vi "AlignTunnelsToControls.vi"(8 "Error In":errorcluster, 10 "New case structure ref":refnum<vi>, 11 "VI ref in":refnum<vi>) -> (0 "Error Out":errorcluster)   [LabVIEW 2017, in "ErrorStructureDrawer.lvlib"]
doc: "Aligns each tunnel on the new case structure to the control/indicator that it is wired to.\n\nNote that the case selector is not aligned by this VI."
uses:
  ErrorStructureDrawer.lvlib
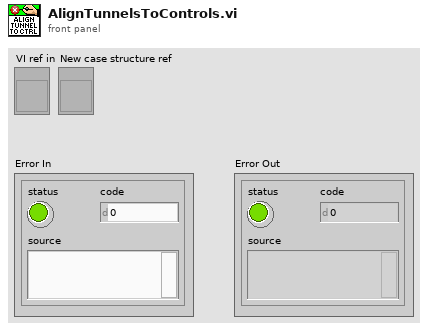
[diagram p1: front panel]
types:
  T1 = enum32{"LooseEnd", "Endpoint", "Bend", "Junction"}
  T2 = typedef "ErrorStructureDrawer.lvlib/ControlConstants.ctl" = cluster{"Half-height of terminal":i32}
  T3 = typedef "ErrorStructureDrawer.lvlib/CaseStructureConstants.ctl" = cluster{"Border thickness":u32, "Case-menu height":u32, "Half height/width of a tunnel":i32}
  T4 = cluster{"Position":cluster{"h":i16, "v":i16}, "Flags":i32, "Type":enum32{"LooseEnd", "Endpoint", "Bend", "Junction"}, "Up Joint Index":i16, "Down Joint Index":i16, "Left Joint Index":i16, "Right Joint Index":i16}[]
  T5 = cluster{"Position":cluster{"h":i16, "v":i16}, "Flags":i32, "Type":enum32{"LooseEnd", "Endpoint", "Bend", "Junction"}, "Up Joint Index":i16, "Down Joint Index":i16, "Left Joint Index":i16, "Right Joint Index":i16}
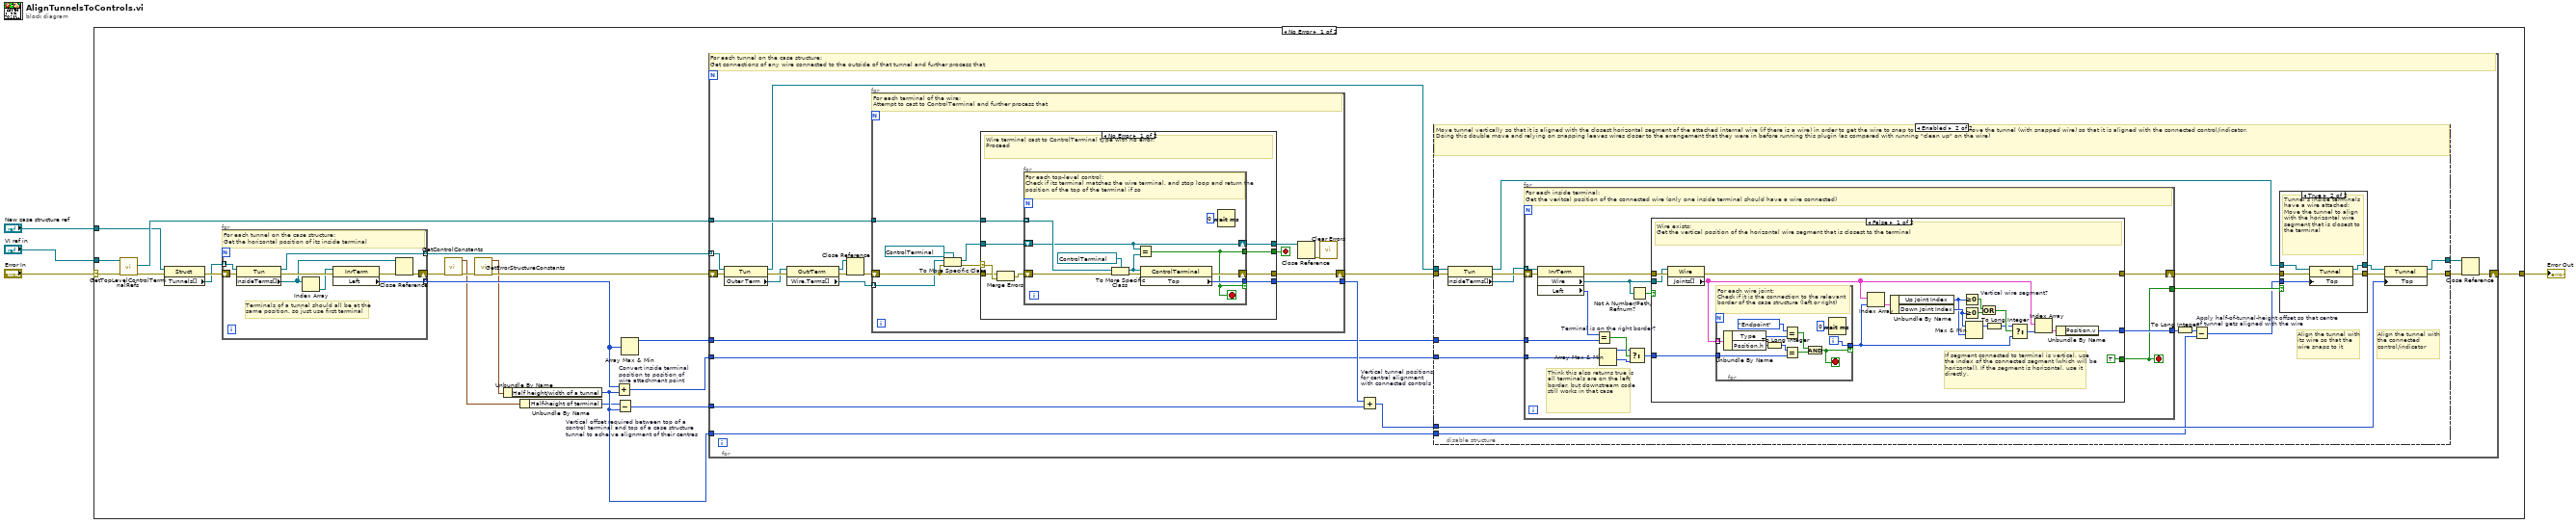
[diagram p0: block diagram]
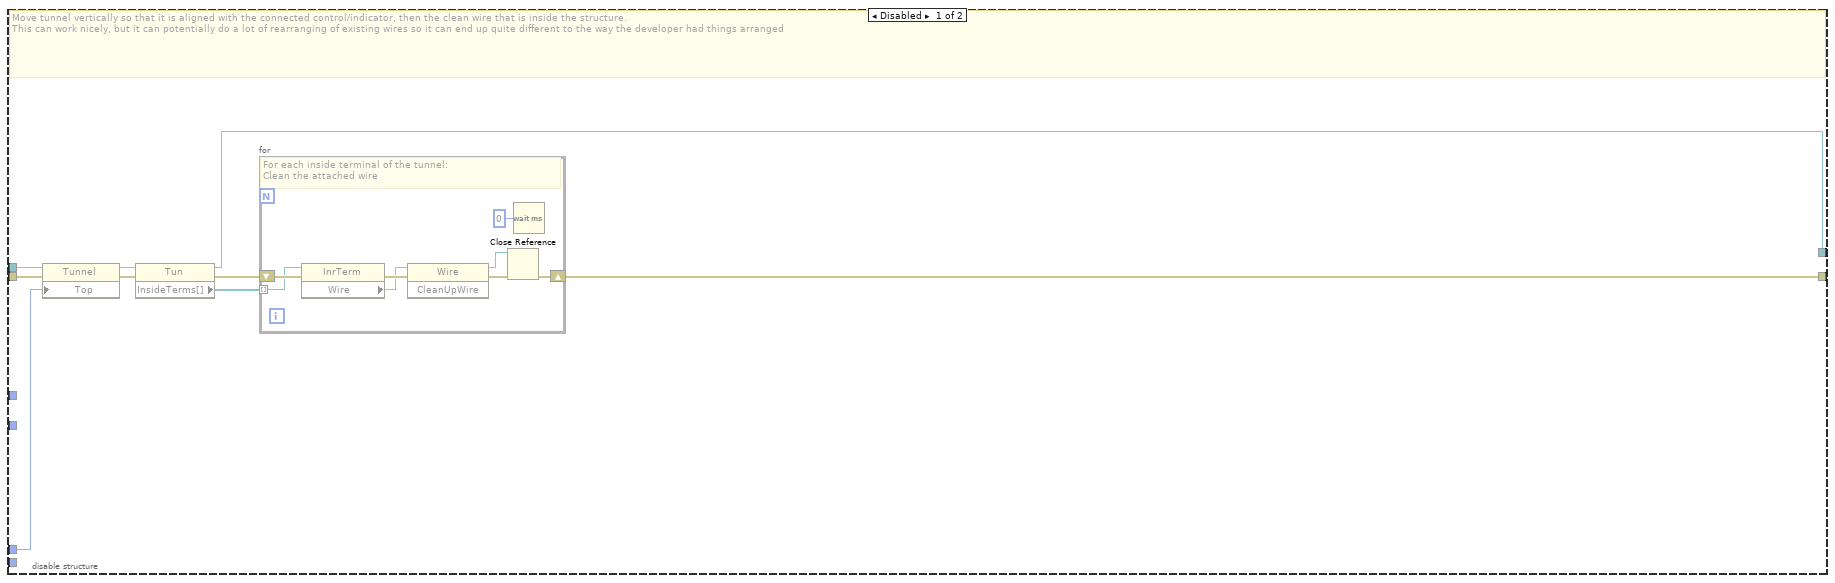
[diagram p2: hidden frame]
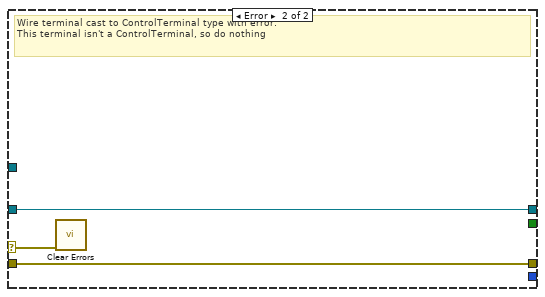
[diagram p5: hidden frame]
diagram:
  n1 = case shown="No Error" "Error In" {
    selector: "Error In" -> [w11 w174]
    tunnel: "VI ref in" -> [w20 _]
    tunnel: "New case structure ref" -> [w19 _]
    tunnel: [w10 w174] -> w1
    frame No Error {
      n2 = call "GetTopLevelControlTerminalRefs.vi"("error in (no error)"=w11, "VI ref in"=w20) -> ("error out"=w18:errorcluster, "Control terminals on top-level"=w21:refnum<vi>[])  [unwired: 7 in, 1 out]
      n3 = property class="Struct"(reference=w19, error in=w18) -> (error out=w22:errorcluster, "Tunnels[]"=w15:refnum<vi>[])  [unwired: 1 out]
      n4 = for {
        tunnel: w15 -> [w172] mode=indexing
        tunnel: [w170] -> w16 mode=indexing
        tunnel: [w169] -> w14 mode=indexing
        shift-right: [w165] -> w5
        shift-left: w22 -> [w168]
        # "Terminals of a tunnel should all be at the same position, so just use first terminal"
        # "For each tunnel on the case structure:\nGet the horizontal position of its inside terminal"
        n5 = property class="Tun"(reference=w172, error in=w168) -> (reference out=w169:refnum<vi>, error out=w173:errorcluster, "InsideTerms[]"=w167:refnum<vi>[])
        n6 = Index Array(array=w167) -> (element=w171:refnum<vi>)  [unwired: 1 in]
        n7 = property class="InrTerm"(reference=w171, error in=w173) -> (error out=w166:errorcluster, "Left"=w170:i32)  [unwired: 1 out]
        n8 = Close Reference(reference=w167, error in (no error)=w166) -> (error out=w165:errorcluster)
      }
      n9 = call "GetControlConstants.vi"("error in (no error)"=w5) -> ("error out"=w24:errorcluster, "Control constants"=w7:T2)  [unwired: 9 in]
      n10 = call "GetErrorStructureConstants.vi"("error in (no error)"=w24) -> ("error out"=w23:errorcluster, "Case structure constants"=w9:T3)  [unwired: 9 in]
      n11 = Unbundle By Name(w9) -> ("Half height/width of a tunnel"=w8:i32)
      n12 = Unbundle By Name(w7) -> ("Half-height of terminal"=w6:i32)
      n13 = Add "Convert inside terminal position to position of wire attachment point"(x=w16, y=w8) -> (x+y=w12:i32[])
      n14 = Subtract "Vertical offset required between top of a control terminal and top of a case structure tunnel to acheive alignment of their centres"(x=w6, y=w8) -> (x-y=w17:i32)
      n15 = Array Max & Min(array=w16) -> (max value=w13:i32)  [unwired: 3 out]
      n16 = for {
        tunnel: w14 -> [w43] mode=indexing
        tunnel: w21 -> [w42]
        shift-right: [w28] -> w10
        shift-left: w23 -> [w39]
        tunnel: w17 -> [w34]
        tunnel: w8 -> [w30]
        tunnel: w13 -> [w26]
        tunnel: w12 -> [w25]
        # "For each tunnel on the case structure:\nGet connections of any wire connected to the outside of that tunnel and further process that"
        n17 = property class="Tun"(reference=w43, error in=w39) -> (reference out=w31:refnum<vi>, error out=w44:errorcluster, "Outer Term"=w41:refnum<vi>)
        n18 = property class="OutrTerm"(reference=w41, error in=w44) -> (reference out=w37:refnum<vi>, error out=w38:errorcluster, "Wire.Terms[]"=w40:refnum<vi>[])
        n19 = Close Reference(reference=w37, error in (no error)=w38) -> (error out=w36:errorcluster)
        n20 = for {
          tunnel: w40 -> [w141] mode=indexing
          tunnel: w42 -> [w140]
          tunnel: [w139] -> w35
          shift-right: [w133] -> w32
          shift-left: w36 -> [w142]
          stop <- w138 stop-if-true
          # "For each terminal of the wire:\nAttempt to cast to ControlTerminal and further process that"
          n21 = To More Specific Class(target class=refnum<vi> refnum ("New case structure ref"), reference=w141, error in=w142) -> (specific class reference=w137:refnum<vi>, error out=w135:errorcluster)
          n22 = case shown="No Error" w135 {
            selector: w135 -> [w151 w162]
            tunnel: w140 -> [w149 _]
            tunnel: [w148 _] -> w139
            tunnel: [w147 _] -> w138
            tunnel: w137 -> [w146 w164]
            tunnel: [w145 w164] -> w134
            tunnel: [w150 w163] -> w133
            tunnel: w142 -> [w144 w163]
            frame No Error {
              # "Wire terminal cast to ControlTerminal type with no error:\nProceed"
              n23 = Merge Errors(w144, w151) -> (w143:errorcluster)
              n24 = for {
                tunnel: w149 -> [w161] mode=indexing
                tunnel: [w159] -> w148 if=w152
                tunnel: [w152] -> w147
                shift-right: [w157] -> w150
                shift-left: w143 -> [w155]
                shift-right: [w153] -> w145
                shift-left: w146 -> [w153]
                stop <- w152 stop-if-true
                # "For each top-level control:\nCheck if its terminal matches the wire terminal, and stop loop and return the position of the top of the terminal if so"
                n25 = To More Specific Class(target class=refnum<vi> refnum ("New case structure ref"), reference=w161, error in=w155) -> (specific class reference=w154:refnum<vi>, error out=w156:errorcluster)
                n26 = Equal?(x=w153, y=w154) -> (x = y?=w152:bool)
                n27 = property class="ControlTerminal"(reference=w154, error in=w156) -> (error out=w157:errorcluster, "Top"=w159:i32)  [unwired: 1 out]
                n28 = Wait (ms)(milliseconds to wait=u32 0) -> ()  [unwired: 1 out]
              }
            }
            frame Error {
              # "Wire terminal cast to ControlTerminal type with error:\nThis terminal isn't a ControlTerminal, so do nothing"
              n29 = call <vilib>:"Clear Errors.vi"("error in (no error)"=w162) -> ()  [unwired: 5 in, 2 out]
            }
          }
          n30 = Close Reference(reference=w134) -> (error out=w132:errorcluster)  [unwired: 1 in]
          n31 = call <vilib>:"Clear Errors.vi"("error in (no error)"=w132) -> ()  [unwired: 5 in, 2 out]
        }
        n32 = Add "Vertical tunnel positions for central alignment with connected controls"(x=w35, y=w34) -> (x+y=w33:i32)
        n33 = disable-structure shown="Enabled" {
          disable-tunnel: w33 -> [w52 w78]
          disable-tunnel: w32 -> [w51 w65]
          disable-tunnel: w31 -> [w47 w70]
          disable-tunnel: [w46 w66] -> w29
          disable-tunnel: [w45 w69] -> w27
          disable-tunnel: w30 -> [_ w77]
          disable-tunnel: w26 -> [_ w68]
          disable-tunnel: w25 -> [_ w67]
          frame Disabled {
            # "Move tunnel vertically so that it is aligned with the connected control/indicator, then the clean wire that is inside the structure.\nThis can work nicely, but it can potentially do a lot of rearranging of existing wires so it can end up quite different to the way the developer had things arranged"
            n34 = property class="Tunnel"(reference=w47, error in=w51, "Top"=w52) -> (reference out=w53:refnum<vi>, error out=w50:errorcluster)
            n35 = property class="Tun"(reference=w53, error in=w50) -> (reference out=w45:refnum<vi>, error out=w49:errorcluster, "InsideTerms[]"=w48:refnum<vi>[])
            n36 = for {
              tunnel: w48 -> [w59] mode=indexing
              shift-right: [w55] -> w46
              shift-left: w49 -> [w60]
              # "For each inside terminal of the tunnel:\nClean the attached wire"
              n37 = property class="InrTerm"(reference=w59, error in=w60) -> (error out=w61:errorcluster, "Wire"=w58:refnum<vi>)  [unwired: 1 out]
              n38 = invoke class="Wire" method="CleanUpWire"(reference=w58, error in=w61) -> (reference out=w54:refnum<vi>, error out=w57:errorcluster)  [unwired: 1 in, 1 out]
              n39 = Close Reference(reference=w54, error in (no error)=w57) -> (error out=w55:errorcluster)
              n40 = Wait (ms)(milliseconds to wait=u32 0) -> ()  [unwired: 1 out]
            }
          }
          frame Enabled {
            # "Align the tunnel with its wire so that the wire snaps to it"
            # "Align the tunnel with the connected control/indicator"
            # "Move tunnel vertically so that it is aligned with the closest horizontal segment of the attached internal wire (if there is a wire) in order to get the wire to snap to the tunnel, then move the tunnel (with snapped wire) so that it is aligned with the connected control/indicator.\nDoing this double move and relying on snapping leaves wires closer to the arrangement that they were in before running this plugin (as compared with running \"clean up\" on the wire)"
            n41 = property class="Tun"(reference=w70, error in=w65) -> (reference out=w73:refnum<vi>, error out=w79:errorcluster, "InsideTerms[]"=w72:refnum<vi>[])
            n42 = for {
              tunnel: w72 -> [w94] mode=indexing
              tunnel: [w93] -> w75
              tunnel: [w90] -> w76
              tunnel: w68 -> [w88]
              tunnel: w67 -> [w87]
              shift-right: [w80] -> w64
              shift-left: w79 -> [w82]
              stop <- w90 stop-if-true
              # "Think this also returns true is all terminals are on the left border, but downstream code still works in that case"
              # "For each inside terminal:\nGet the veritcal position of the connected wire (only one inside terminal should have a wire connected)"
              n43 = property class="InrTerm"(reference=w94, error in=w82) -> (error out=w81:errorcluster, "Wire"=w92:refnum<vi>, "Left"=w89:i32)  [unwired: 1 out]
              n44 = Equal? "Terminal is on the right border?"(x=w89, y=w88) -> (x = y?=w86:bool)
              n45 = Array Max & Min(array=w87) -> (max value=w85:i32, min value=w84:i32)  [unwired: 2 out]
              n46 = Select(t=w85, s=w86, f=w84) -> (s? t:f=w83:i32)
              n47 = Not A Number/Path/Refnum?(number/path/refnum=w92) -> (NaN/Path/Refnum?=w91:bool)
              n48 = case shown="False" w91 {
                tunnel: [TRUE _] -> w90
                tunnel: [w103 _] -> w93
                tunnel: w92 -> [w111 _]
                tunnel: w83 -> [w98 _]
                tunnel: w81 -> [w112 w124]
                tunnel: [w96 w124] -> w80
                frame False {
                  # "If segment connected to terminal is vertical, use the index of the connected segment (which will be horizontal). If the segment is horizontal, use it directly."
                  # "Wire exists:\nGet the vertical position of the horizontal wire segment that is closest to the terminal"
                  n49 = property class="Wire"(reference=w111, error in=w112) -> (error out=w96:errorcluster, "Joints[]"=w99:T4)  [unwired: 1 out]
                  n50 = for {
                    tunnel: w99 -> [w123] mode=indexing
                    tunnel: w98 -> [w122]
                    tunnel: [w117] -> w97 if=w116
                    i -> [w117]
                    stop <- w116 stop-if-true
                    # "For each wire joint:\nCheck if it is the connection to the relevant border of the case structure (left or right)"
                    n51 = Unbundle By Name(w123) -> ("Type"=w121:T1, "Position.h"=w115:i16)
                    n52 = To Long Integer(number=w115) -> (32bit integer=w114:i32)
                    n53 = Equal?(x=T1."Endpoint", y=w121) -> (x = y?=w119:bool)
                    n54 = Equal?(x=w114, y=w122) -> (x = y?=w118:bool)
                    n55 = And(x=w119, y=w118) -> (x .and. y?=w116:bool)
                    n56 = Wait (ms)(milliseconds to wait=u32 0) -> ()  [unwired: 1 out]
                  }
                  n57 = Index Array(array=w99, index=w97) -> (element=w110:T5)
                  n58 = Unbundle By Name(w110) -> ("Up Joint Index"=w100:i16, "Down Joint Index"=w101:i16)
                  n59 = Greater Or Equal To 0?(x=w100) -> (x >= 0?=w109:bool)
                  n60 = Greater Or Equal To 0?(x=w101) -> (x >= 0?=w108:bool)
                  n61 = Max & Min(x=w101, y=w100) -> (max(x,y)=w106:i16)  [unwired: 1 out]
                  n62 = Or "Vertical wire segment?"(x=w109, y=w108) -> (x .or. y?=w107:bool)
                  n63 = To Long Integer(number=w106) -> (32bit integer=w95:i32)
                  n64 = Select(t=w95, s=w107, f=w97) -> (s? t:f=w105:i32)
                  n65 = Index Array(array=w99, index=w105) -> (element=w104:T5)
                  n66 = Unbundle By Name(w104) -> ("Position.v"=w103:i16)
                }
                frame True {
                  # "Wire doesn't exist:\nDo nothing"
                }
              }
            }
            n67 = To Long Integer(number=w75) -> (32bit integer=w62:i32)
            n68 = Subtract "Apply half-of-tunnel-height offset so that centre of tunnel gets aligned with the wire"(x=w62, y=w77) -> (x-y=w74:i32)
            n69 = case shown="True" w76 {
              tunnel: w73 -> [w126 w129]
              tunnel: w74 -> [_ w128]
              tunnel: [w126 w127] -> w71
              tunnel: w64 -> [w125 w130]
              tunnel: [w125 w131] -> w63
              frame False {
                # "Tunnel's inside terminals have no wire attached:\nDo nothing"
              }
              frame True {
                # "Tunnel's inside terminals have a wire attached:\nMove the tunnel to align with the horizontal wire segment that is closest to the terminal"
                n70 = property class="Tunnel"(reference=w129, error in=w130, "Top"=w128) -> (reference out=w127:refnum<vi>, error out=w131:errorcluster)
              }
            }
            n71 = property class="Tunnel"(reference=w71, error in=w63, "Top"=w78) -> (reference out=w69:refnum<vi>, error out=w66:errorcluster)
          }
        }
        n72 = Close Reference(reference=w27, error in (no error)=w29) -> (error out=w28:errorcluster)
      }
    }
    frame Error {
    }
  }
  "Error Out" <- w1
